vi "I.vi"(9 "Z":u32 format="%08x", 10 "Y":u32 format="%08x", 11 "X":u32 format="%08x") -> (3 "I":u32 format="%08x")   [LabVIEW 2013, in "MD5.lvlib" / "MD5.lvclass"]
uses:
  MD5.lvclass
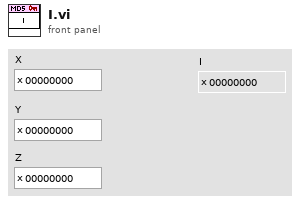
[diagram p1: front panel]
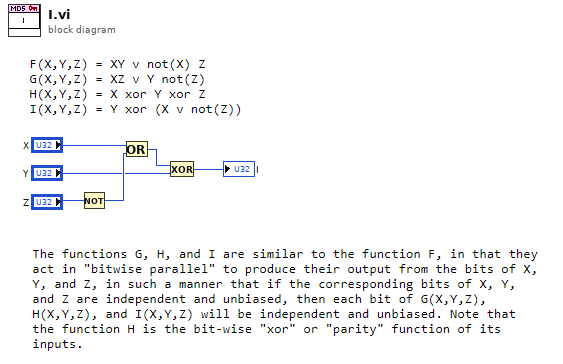
[diagram p0: block diagram]
diagram:
  n1 = Not(x="Z") -> (.not. x?=w6:u32)
  n2 = Or(x="X", y=w6) -> (x .or. y?=w3:u32)
  n3 = Exclusive Or(1:"Y", 2:w3) -> (0:→"I":u32)
